vi "Convert Dictionary to ITEMs and VALUEs.vi"(8 "error in (no error)":errorcluster, 11 "Data (Dictionary)":T1[](array[typedef])) -> (0 "error out":errorcluster, 1 "2D Array of Variants":variant[][](array[variant]), 2 "ITEMS":string[](array[string]), 3 "Data (Dictionary)":T1[](array[typedef]))   [LabVIEW 2020, in "Data.PG.lvclass"]
uses:
  Data.PG.lvclass
  Data/Typedefs/Dictionary--cluster.ctl
  Data/Data.lvclass
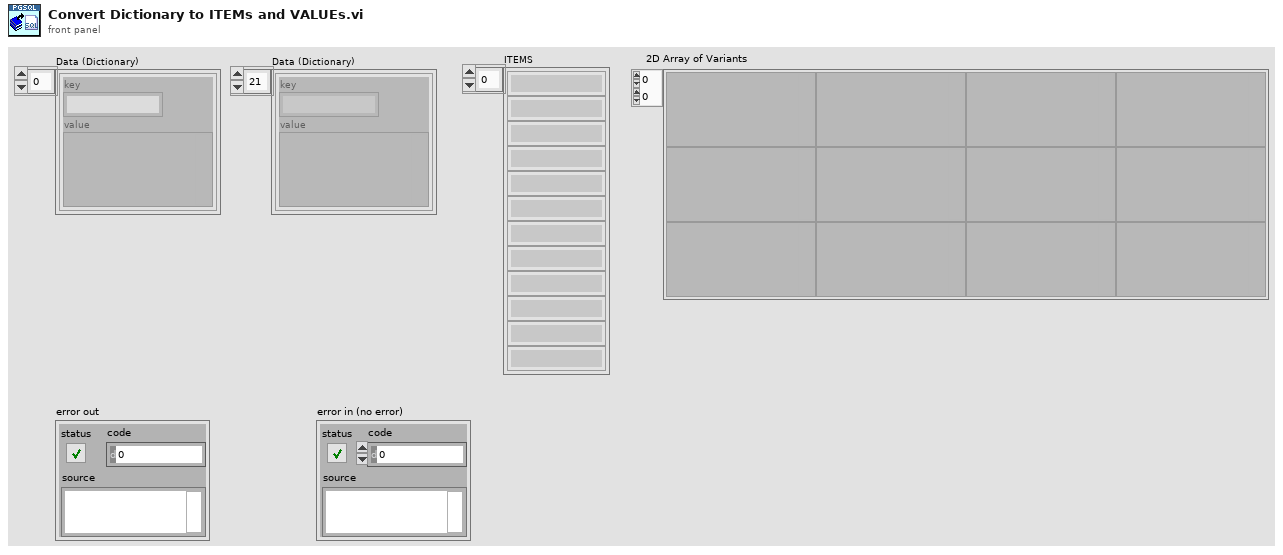
[diagram p1: front panel]
types:
  T1 = typedef "Data.lvclass/Dictionary--cluster.ctl" = cluster{"key":string, "value":variant}
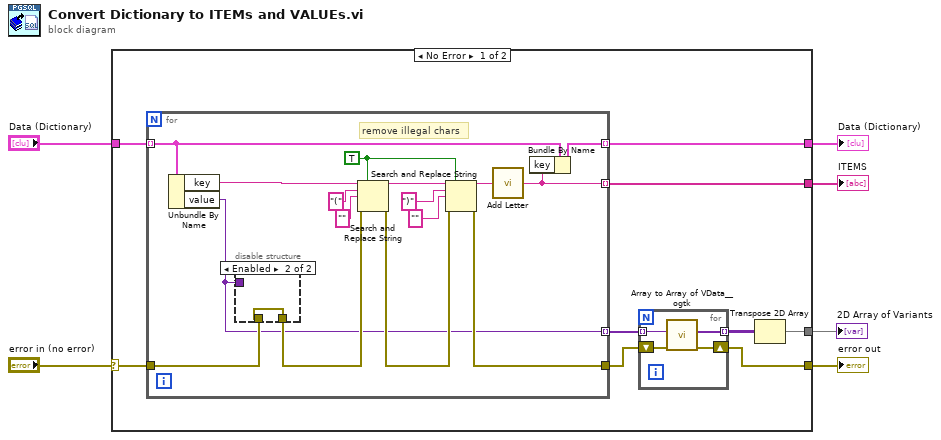
[diagram p0: block diagram]
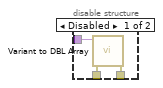
[diagram p2: hidden frame]
diagram:
  n1 = case shown="No Error" "error in (no error)" {
    selector: "error in (no error)" -> [w14 w40]
    tunnel: [w7 w40] -> w6
    tunnel: "Data (Dictionary)" -> [w15 _]
    tunnel: [w13 _] -> w3
    tunnel: [w12 _] -> w2
    tunnel: [w9 _] -> w1
    frame No Error {
      n2 = for {
        tunnel: w15 -> [w20] mode=indexing
        tunnel: w14 -> [w29]
        tunnel: [w19] -> w8
        tunnel: [w21] -> w13 mode=indexing
        tunnel: [w16] -> w12 mode=indexing
        tunnel: [w18] -> w10 mode=indexing
        w24 = TRUE ("replace all? (F)")
        # "remove illegal chars"
        n3 = Unbundle By Name(w20) -> ("key"=w30:string, "value"=w18:variant)
        n4 = disable-structure shown="Enabled" {
          disable-tunnel: w29 -> [w34 w35]
          disable-tunnel: [w33 w35] -> w23
          disable-tunnel: w18 -> [w32 _]
          frame Disabled {
            n5 = call "Variant to DBL Array.vi"("error in (no error)"=w34, "Data (Variant)"=w32) -> ("error out"=w33:errorcluster)  [unwired: 7 in, 2 out]
          }
          frame Enabled {
          }
        }
        n6 = Search and Replace String(replace all?=w24, input string=w30, search string="(", replace string="" ("replace string (\"\")"), error in=w23) -> (result string=w25:string, error out=w22:errorcluster)  [unwired: 3 in, 2 out]
        n7 = Search and Replace String(replace all?=w24, input string=w25, search string=")", replace string="" ("replace string (\"\")"), error in=w22) -> (result string=w17:string, error out=w19:errorcluster)  [unwired: 3 in, 2 out]
        n8 = call "Add Letter.vi"("string"=w17) -> ("result string"=w16:string)
        n9 = Bundle By Name(cluster=w20, "key"=w16) -> (w21:T1)
      }
      n10 = for {
        tunnel: [w39] -> w11 mode=indexing
        tunnel: w10 -> [w38] mode=indexing
        shift-right: [w36] -> w7
        shift-left: w8 -> [w37]
        n11 = call <userlib>:"Array to Array of VData__ogtk.vi"("error in (no error)"=w37, "MultiD Array"=w38) -> ("error out"=w36:errorcluster, "1D Array of Variants"=w39:variant[])  [unwired: 8 in]
      }
      n12 = Transpose 2D Array(2D array=w11) -> (transposed array=w9:variant[][])
    }
    frame Error {
    }
  }
  "ITEMS" <- w2
  "error out" <- w6
  "Data (Dictionary)" <- w3
  "2D Array of Variants" <- w1
